vi "MicroPulse - decode voltage sets.vi"(0 "U8":u8[](array[numeric])) -> (2 "voltages":string, 3 "Voltages":T1(array[cluster]) {"Difference" format="%.2fV"; "Measured" format="%.2fV"; "Nominal" format="%.2fV"})   [LabVIEW 2026, in "MicroPulse_Driver.lvlib"]
uses:
  MicroPulse_Driver.lvlib
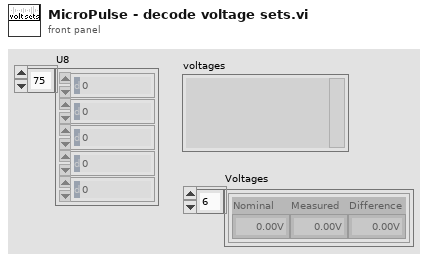
[diagram p1: front panel]
types:
  T1 = cluster{"Nominal":dbl, "Measured":dbl, "Difference":dbl}[]
  T2 = cluster{"voltage setting":dbl, "volts read":dbl, dbl}
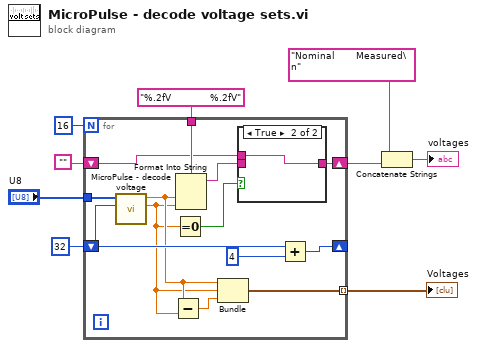
[diagram p0: block diagram]
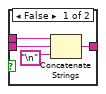
[diagram p2: hidden frame]
diagram:
  n1 = for {
    N: 16 -> [_]
    shift-right: [w21] -> _
    shift-left: 32 ("index") -> [w22]
    tunnel: "U8" -> [w19]
    tunnel: "%.2fV             %.2fV" ("format string") -> [w18]
    shift-right: [w16] -> w4
    shift-left: "" -> [w15]
    tunnel: [w12] -> w1 mode=indexing
    n2 = call "MicroPulse - decode voltage.vi"("start index"=w22, "voltage bytes"=w19) -> ("volts read"=w11:dbl, "voltage setting"=w13:dbl)  [unwired: 4 in]
    n3 = Subtract(x=w13, y=w11) -> (x-y=w14:dbl)
    n4 = Equal To 0?(x=w11) -> (x = 0?=w10:bool)
    n5 = Format Into String(format string=w18, w13, w11) -> (resulting string=w17:string)  [unwired: 2 in, 1 out]
    n6 = Bundle("voltage setting"=w13, "volts read"=w11, w14) -> (w12:T2)  [unwired: 1 in]
    n7 = case shown="True" w10 {
      tunnel: w17 -> [w25 _]
      tunnel: [w24 w27] -> w16
      tunnel: w15 -> [w23 w27]
      frame False {
        n8 = Concatenate Strings(w23, w25, "\n") -> (w24:string)
      }
      frame True {
      }
    }
    n9 = Add(x=w22, y=4) -> (x+y=w21:i32)
  }
  "Voltages" <- w1
  n10 = Concatenate Strings("Nominal       Measured\n" ("format string"), w4) -> (→"voltages":string)
